vi "grSim Packet Command Serial Test.vi"() -> ()   [LabVIEW 2016]
uses:
  grSim/grSim Robot Command.ctl
panel:
  out "return count":u32
  out "error out 2":errorcluster
  in  "VISA Open timeout (0)":u32=500
  in  "VISA resource name":refnum<visa-resource-name>
  out "Array":u8[](array[numeric]) format="%02x"
  in  "isteamyellow":bool=TRUE
  in  "Robots":T1[](array[typedef])
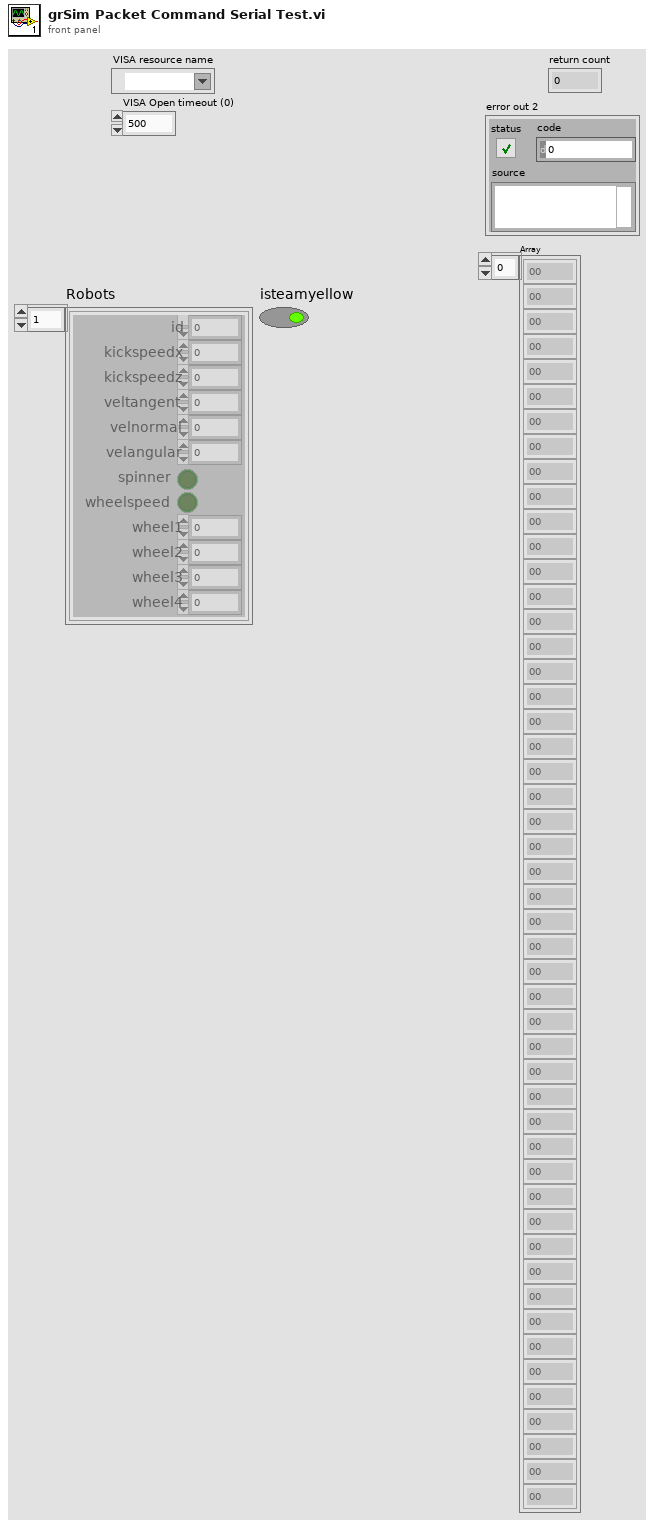
[diagram p1: front panel]
types:
  T1 = typedef "grSim Robot Command.ctl" = cluster{"id":u32, "kickspeedx":sgl, "kickspeedz":sgl, "veltangent":sgl, "velnormal":sgl, "velangular":sgl, "spinner":bool, "wheelspeed":bool, "wheel1":sgl, "wheel2":sgl, "wheel3":sgl, "wheel4":sgl}
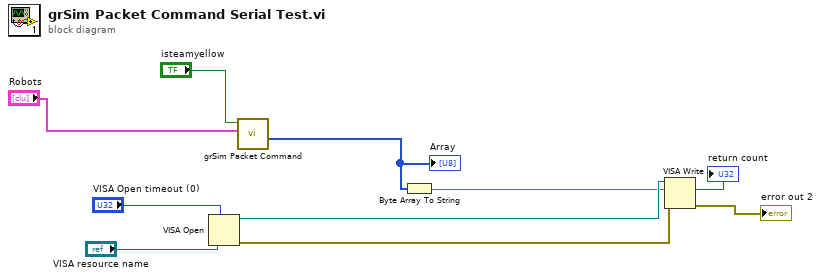
[diagram p0: block diagram]
diagram:
  n1 = VISA Open(timeout (0)="VISA Open timeout (0)", VISA resource name="VISA resource name") -> (VISA resource name=w4:refnum<visa-resource-name>, error out=w3:errorcluster)  [unwired: 3 in]
  n2 = call "grSim Packet Command.vi"("Robots"="Robots", "isteamyellow"="isteamyellow") -> ("Array"=w9:u8[])  [unwired: 9 in]
  "Array" <- w9
  n3 = Byte Array To String(unsigned byte array=w9) -> (string=w2:string)
  n4 = VISA Write(VISA resource name=w4, write buffer=w2, error in (no error)=w3) -> (return count=→"return count":u32, error out=→"error out 2":errorcluster)  [unwired: 1 out]
